vi "New Results (to override).vi"(7 "Image Nr.":i32, 8 "error in (no error)":errorcluster, 9 "Results In":refnum<class "Analyze Results Base.lvclass">[](array[class]), 10 "Parameters":refnum<class "Analyze Parameter Base.lvclass">[](array[class]), 11 "HIJ Single Cam App Demo In":refnum<class "HIJ Vision Camera App w Timer.lvclass">) -> (0 "error out":errorcluster, 3 "HIJ Single Cam App Demo Out":refnum<class "HIJ Vision Camera App w Timer.lvclass">)   [LabVIEW 2014, in "HIJ Vision Camera App w Timer.lvlib" / "HIJ Vision Camera App w Timer.lvclass"]
uses:
  HIJ Vision Camera App w Timer.lvclass
  Analyze/Results and Overlays/Results Base/Analyze Results Base.lvclass
  Analyze/Analyze Parameter/Analyze Parameter Base/Analyze Parameter Base.lvclass
  <vilib>/ActorFramework/Time-Delayed Send Message/Time-Delay Override Options.ctl
  <vilib>/ActorFramework/Actor/Actor.lvclass/Actor.ctl
  HIJ Vision Camera App w Timer.lvclass/HIJ Vision Camera App w Timer.ctl
  Abstract Messages/Publish Analyze Results Msg/Publish Analyze Results Msg.lvclass/Publish Analyze Results Msg.ctl
  <vilib>/ActorFramework/Message Enqueuer/Message Enqueuer.lvclass/Message Enqueuer.ctl
  <vilib>/ActorFramework/Message Enqueuer/Enqueue.vi
  <vilib>/ActorFramework/Message Priority Queue/Priority Enqueue.vi
  <vilib>/ActorFramework/Message Enqueuer/Message Enqueuer.lvclass
  Applications/HIJ Vision Camera App/HIJ Vision Camera App/HIJ Vision Camera App.lvclass
  <vilib>/ActorFramework/Actor/Actor.lvclass
  Abstract Messages/Publish Analyze Results Msg/Publish Analyze Results Msg.lvclass
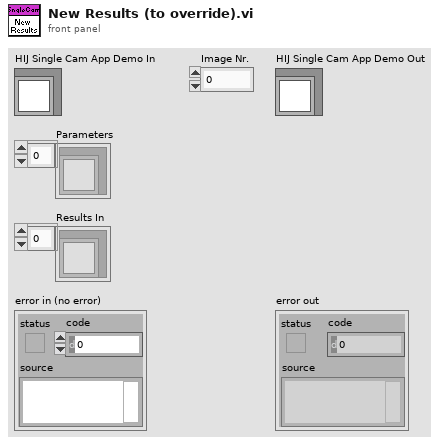
[diagram p1: front panel]
types:
  T1 = typedef "Time-Delay Override Options.ctl" = enum16{"Send next copy now", "Skip next scheduled copy", "Send next copy now and stop all further copies", "Stop all further copies"}
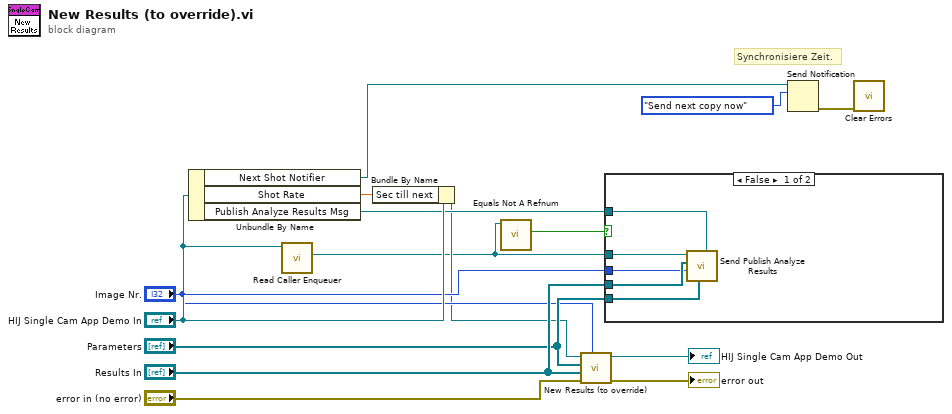
[diagram p0: block diagram]
diagram:
  # "Synchronisiere Zeit."
  n1 = Unbundle By Name("HIJ Single Cam App Demo In") -> ("Next Shot Notifier"=w4:refnum<notifier>, "Shot Rate"=w2:dbl, "Publish Analyze Results Msg"=w11:refnum<class "Publish Analyze Results Msg.lvclass">)
  n2 = call <vilib>:"Read Caller Enqueuer.vi"("Actor"="HIJ Single Cam App Demo In") -> ("Caller Enqueuer"=w1:refnum<class "Message Enqueuer.lvclass">)  [unwired: 10 in]
  n3 = Bundle By Name(cluster="HIJ Single Cam App Demo In", "Sec till next"=w2) -> (w3:refnum<class "HIJ Vision Camera App w Timer.lvclass">)
  n4 = call <vilib>:"Equals Not A Refnum.vi"("Message Enqueuer"=w1) -> ("Not a refnum?"=w8:bool)  [unwired: 10 in]
  n5 = call-parent "New Results (to override).vi"("Image Nr."="Image Nr.", "error in (no error)"="error in (no error)", "Results In"="Results In", "Parameters"="Parameters", "HIJ Vision Camera App In"=w3) -> ("error out"=→"error out":errorcluster, "HIJ Vision Camera App Out"=→"HIJ Single Cam App Demo Out":refnum<class "HIJ Vision Camera App w Timer.lvclass">)  [unwired: 5 in]
  n6 = case shown="False" w8 {
    tunnel: w11 -> [w20 _]
    tunnel: "Results In" -> [w19 _]
    tunnel: "Parameters" -> [w18 _]
    tunnel: w1 -> [w17 _]
    tunnel: "Image Nr." -> [w16 _]
    frame False {
      n7 = call "Send Publish Analyze Results.vi"("Message Type"=w20, "Parameters"=w18, "Image Nr."=w16, "Results In"=w19, "Message Enqueuer"=w17) -> ()  [unwired: 5 in, 2 out]
    }
    frame True {
    }
  }
  n8 = Send Notification(notification=Time-Delay_Override_Options."Send next copy now", notifier=w4) -> (error out=w6:errorcluster)  [unwired: 1 in, 1 out]
  n9 = call <vilib>:"Clear Errors.vi"("error in (no error)"=w6) -> ()  [unwired: 5 in, 2 out]
